vi "Measurement UI.vi"() -> ()   [LabVIEW 2021]
uses:
  bhava/source/shared/controls/PCM Interface Type_Copy.ctl
  bhava/source/shared/controls/Audio ADC Controls.lvlib
  <vilib>/PDM Acquisition Toolkit/shared/controls/Digital Edge.ctl
  <vilib>/PDM Acquisition Toolkit/shared/PDM Shared.lvlib
  bhava/source/shared/Audio ADC Shared.lvlib
panel:
  in  "MeasGraphs":T1(tab)=enum."Time Domain"
  out "FreqDomainGraph":cluster{"f0":dbl, "df":dbl, "Spectrum":dbl[]}[](graph) caption="AC"
  out "TimeDomainGraph":waveform(dbl)[](graph) caption="AC"
  out "Spectrum":dbl[](array[numeric])
  out "df":dbl[](array[numeric])
  out "f0":dbl[](array[numeric])
  out "Time domain":dbl[](array[numeric])
  out "dt":dbl[](array[numeric])
  out "t0":dbl[](array[numeric])
  out "SFDR":dbl[](array[numeric])
  out "Gain error":dbl[](array[numeric])
  out "Dynamic range":dbl[](array[numeric])
  out "THD":dbl[](array[numeric])
  out "THD+N":dbl[](array[numeric])
  out "SNR":dbl[](array[numeric])
  out "Calculated amplitude":dbl[](array[numeric])
  out "Calculated frequency":dbl[](array[numeric])
  out "MeasTable":string[][](table)
  in  "Configuration tab":enum32{"Protocol", "Measurement"}(tab)=enum."Measurement"
  in  "Endianness":enum32{"MSB First", "LSB First"}(ring)
  in  "Bit clock edge  sync":enum32{"Rising", "Falling"}(ring)=enum."Falling"
  in  "Frame sync edge for Channel 0":enum32{"Rising", "Falling"}(ring)=enum."Falling"
  in  "Channel count per frame":u32=2
  in  "Channel length":u32=32
  in  "Bit depth":u32=24
  in  "Channel 0 offset":u32=1
  in  "Data Justification":enum32{"Left Justified", "Right Justified"}(ring) caption="Data justification"
  in  "Frame length":u32=64
  in  "Frame sync pulse width":u32=32
  in  "I2S":bool
  in  "LJ":bool
  in  "RJ":bool
  in  "TDM":bool
  in  "Band stop":dbl=20000.0 format="%#.6pHz"
  in  "Band start":dbl=20.0 format="%#.6pHz"
  in  "Right channel analog source resource name":string(combo) caption="Right channel resource name"
  in  "Protocol capture resource name":string(combo) caption="Resource name"
  in  "Measurement Duration":dbl=0.1 caption="Measurement duration" format="%#_6ps"
  in  "Left channel analog source resource name":string(combo) caption="Left channel resource name"
  in  "Channel name":string
  in  "Full scale range":dbl=2.825 caption="FULL SCALE RANGE" format="%.3pV"
  in  "Weighting Filter":string(combo)="Linear" caption="Weighting filter"
  in  "Data line":u32
  in  "Sample rate":dbl=44100.0 format="%#.6pHz"
  in  "Measurement settings":string="Measurement Settings"
  in  "Amplitude":dbl=-1.0 format="%#_6pdB"
  in  "Frequency":dbl=1000.0 format="%#_6pHz"
  in  "Right acquisition channel":u32=1
  in  "Left acquisition channel":u32
  in  "Analog source":string="Analog source"
  in  "Digital capture":string="Digital capture"
  # "Protocols"
  # "PCM data configuration"
  # "Frame sync clock control"
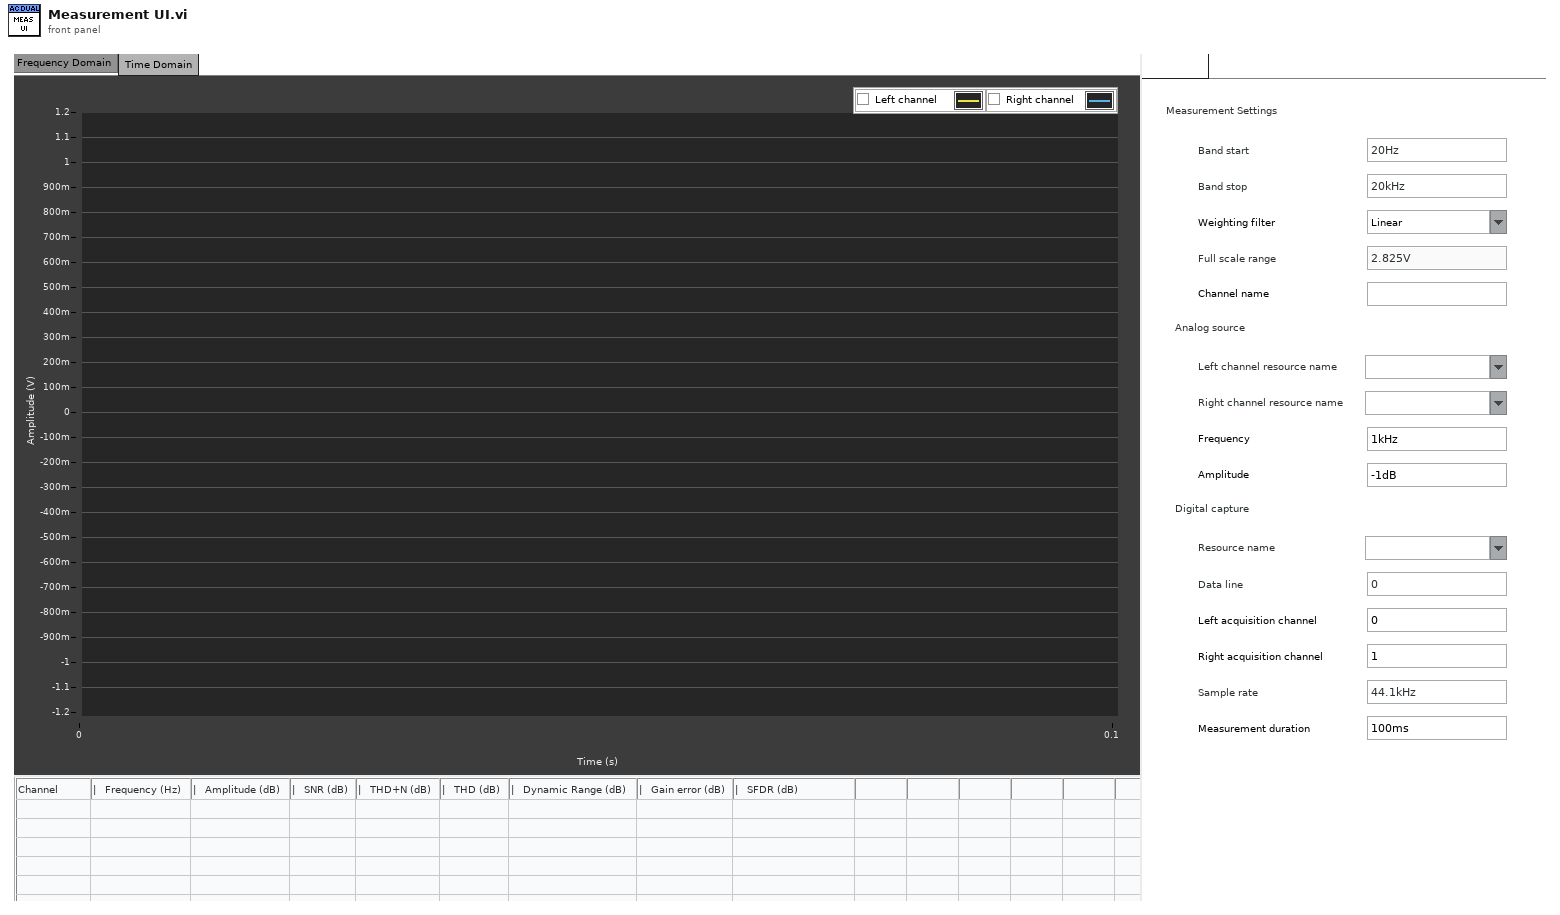
[diagram p1: front panel]
types:
  T1 = enum32{"Frequency Domain", "Time Domain", "Hidden Controls"}
  T2 = typedef "PDM Shared.lvlib/Digital Edge.ctl" = enum8{"Rising", "Falling"}
  T3 = typedef "Audio ADC Controls.lvlib/PCM Interface Type_Copy.ctl" = enum16{"I2S", "Left Justified", "Right Justified", "TDM 4 Channel", "TDM 6 Channel", "TDM 8 Channel", "DSP mode", "DSP mode with 1 bit delay", "PCM Short Frame", "PCM Long Frame"}
  T4 = typedef "PDM Shared.lvlib/PCM Frame Sync Control.ctl" = cluster{"Frame Length":u16, "Frame Sync Pulse Width":u16, "Bit Clock Edge  Sync":T2}
  T5 = typedef "PDM Shared.lvlib/PCM Data Format Configuration.ctl" = cluster{"Frame Sync Edge for Channel 0":T2, "Channel Count Per Frame":u8, "Channel Length":u16, "Bit Depth":u8, "Channel 0 Offset":u16, "Endianness":T6, "Data Justification":T7}
  T6 = typedef "PDM Shared.lvlib/PCM Bit Endianness.ctl" = enum16{"MSB First", "LSB First"}
  T7 = typedef "PDM Shared.lvlib/PCM Data Justification.ctl" = enum16{"Left Justified", "Right Justified"}
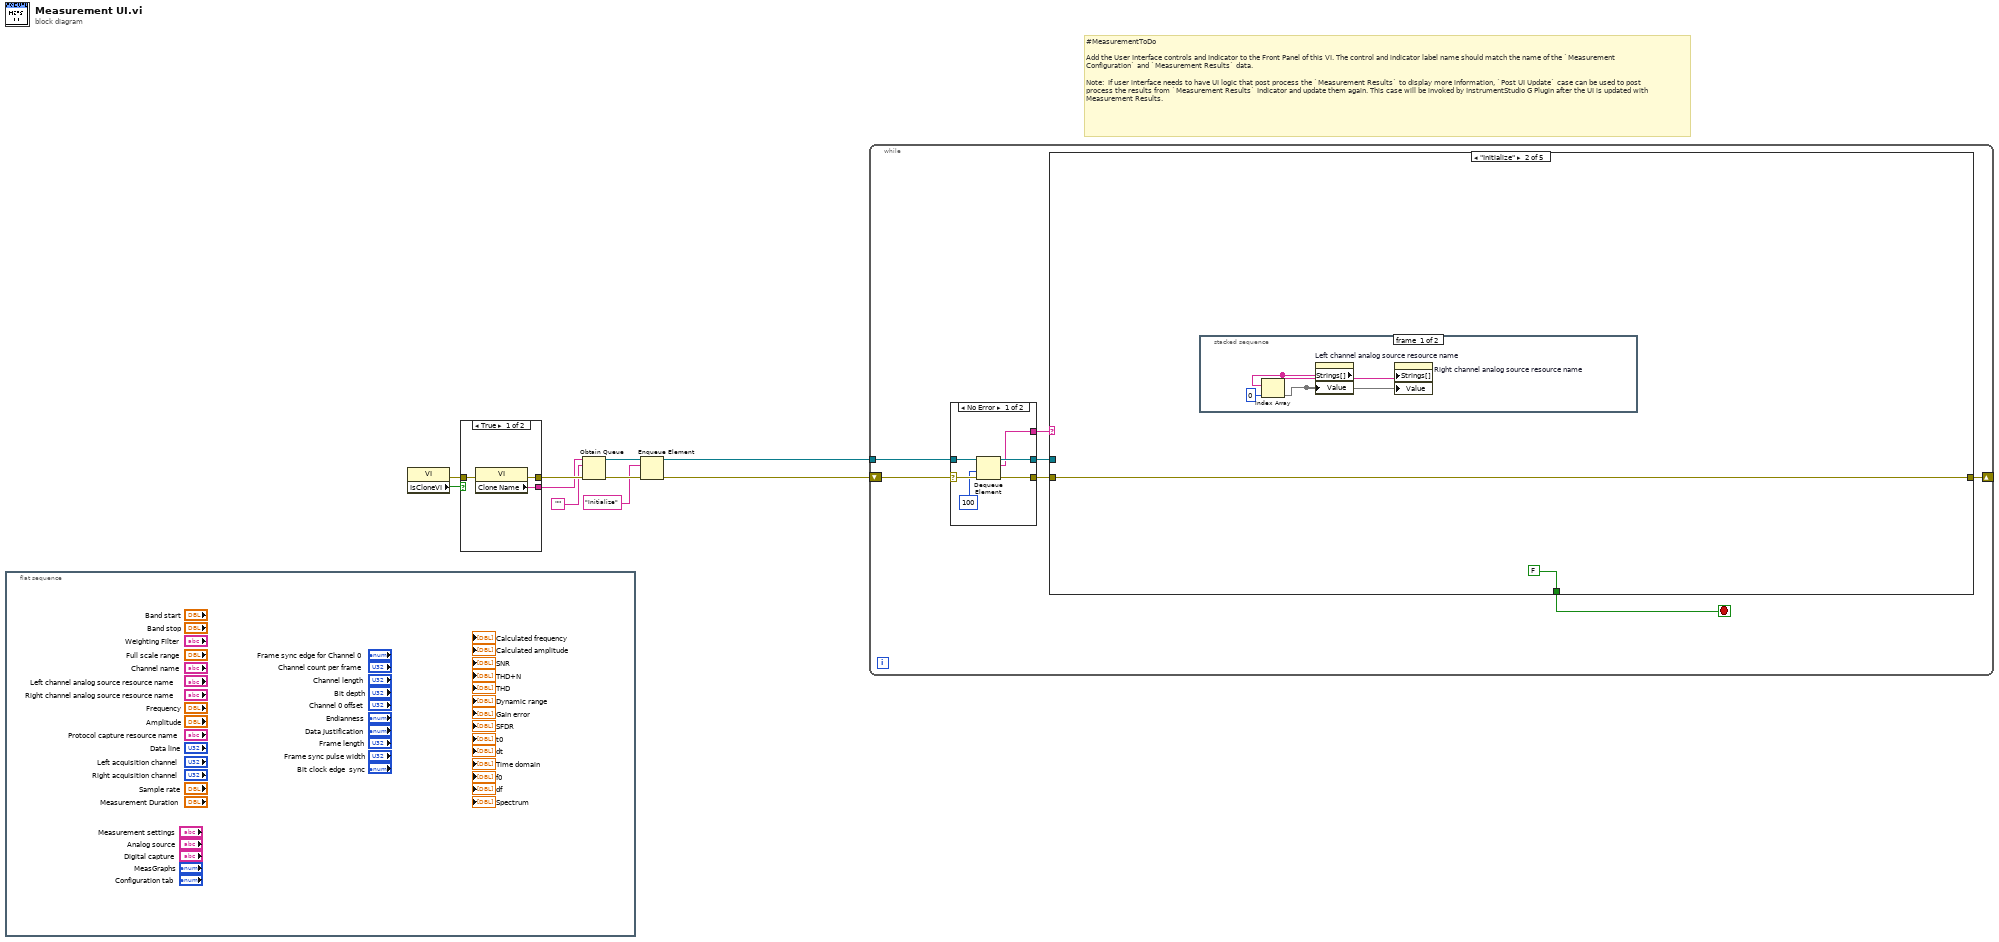
[diagram p0: block diagram]
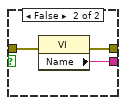
[diagram p2: hidden frame]
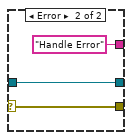
[diagram p3: hidden frame]
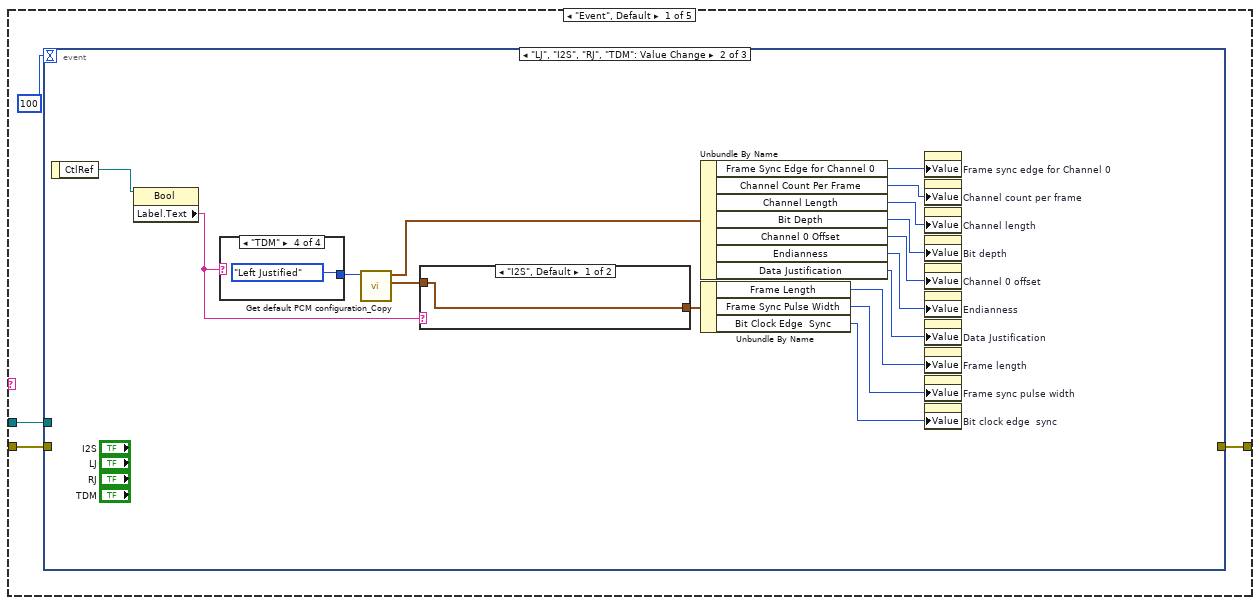
[diagram p4: hidden frame]
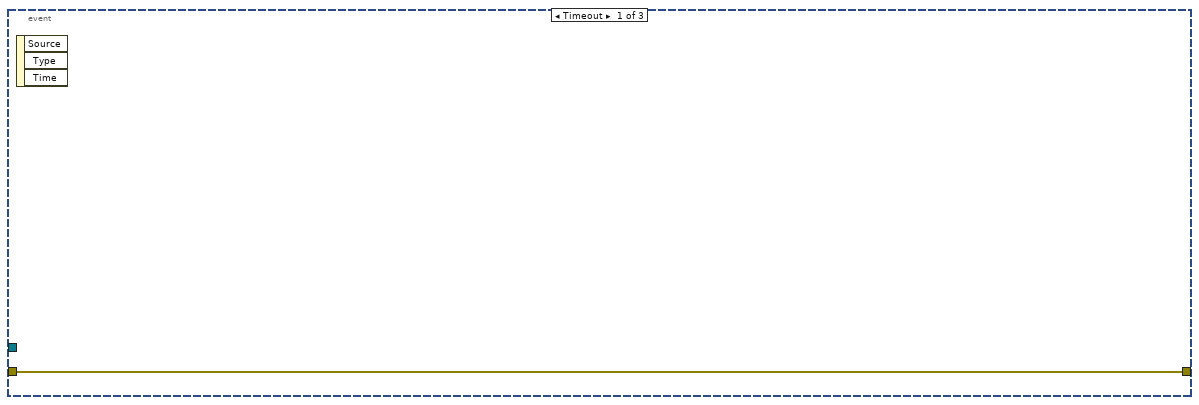
[diagram p5: hidden frame]
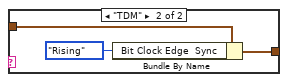
[diagram p6: hidden frame]
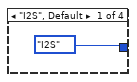
[diagram p7: hidden frame]
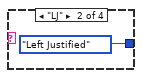
[diagram p8: hidden frame]
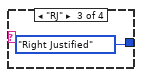
[diagram p9: hidden frame]
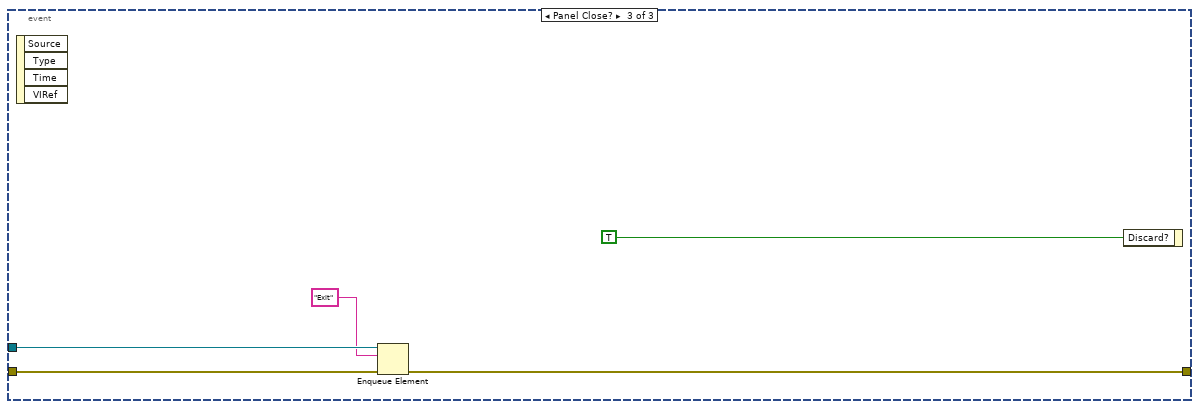
[diagram p10: hidden frame]
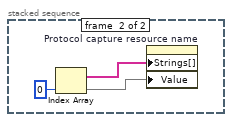
[diagram p11: hidden frame]
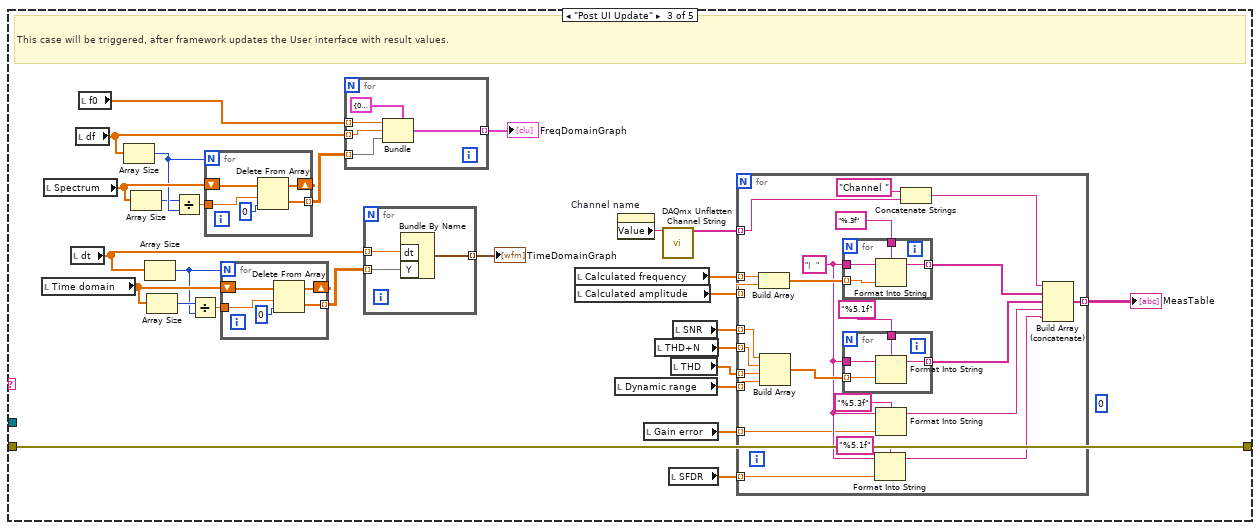
[diagram p12: hidden frame]
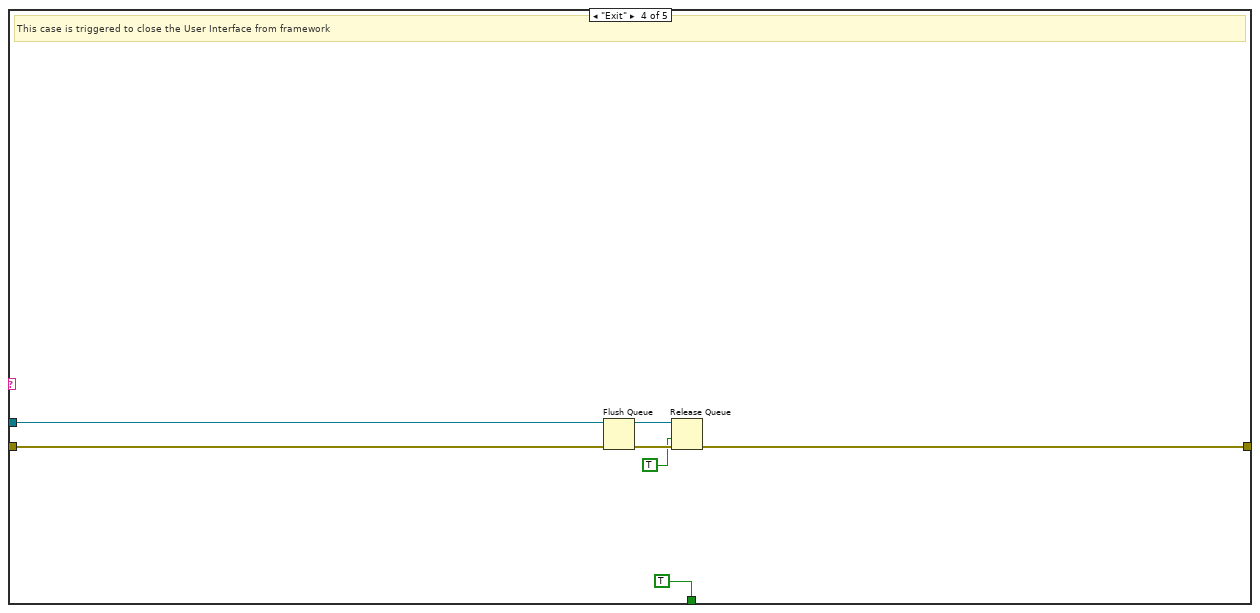
[diagram p13: hidden frame]
diagram:
  # "#MeasurementToDo  \n\nAdd the User Interface controls and Indicator to the Front Panel of this VI. The control and indicator label name should match the name of the `Measurement Configuration` and `Measurement Results` data.\n\nNote:  If user interface needs to have UI logic that post process the `Measurement Results` to display more information, `Post UI Update` case can be used to post process the results from `Measurement Results` Indicator and update them again. This case will be invoked by InstrumentStudio G Plugin after the UI is updated with Measurement Results."
  n1 = flat-sequence {
    frame #0 {
    }
  }
  n2 = property class="VI"() -> (error out=w1:errorcluster, "IsCloneVI"=w2:bool)  [unwired: 2 in, 1 out]
  n3 = case shown="True" w2 {
    tunnel: [w13 w16] -> w10
    tunnel: [w12 w15] -> w9
    tunnel: w1 -> [w11 w14]
    frame True {
      n4 = property class="VI"(error in=w11) -> (error out=w13:errorcluster, "Clone Name"=w12:string)  [unwired: 1 in, 1 out]
    }
    frame False {
      n5 = property class="VI"(error in=w14) -> (error out=w16:errorcluster, "Name"=w15:string)  [unwired: 1 in, 1 out]
    }
  }
  n6 = Obtain Queue(name (unnamed)=w9, element data type="", error in (no error)=w10) -> (queue out=w6:refnum<queue>, error out=w8:errorcluster)  [unwired: 2 in, 1 out]
  n7 = Enqueue Element(queue=w6, element="Initialize", error in (no error)=w8) -> (queue out=w5:refnum<queue>, error out=w7:errorcluster)  [unwired: 1 in, 1 out]
  n8 = while {
    shift-right: [w18] -> _
    shift-left: w7 -> [w23]
    tunnel: w5 -> [w21]
    stop <- w17 stop-if-true
    n9 = case shown="No Error" w23 {
      selector: w23 -> [w29 w32]
      tunnel: [w28 w32] -> w22
      tunnel: w21 -> [w27 w31]
      tunnel: [w26 w31] -> w20
      tunnel: [w25 "Handle Error"] -> w19
      frame No Error {
        n10 = Dequeue Element(queue=w27, timeout in ms (-1)=100, error in (no error)=w29) -> (queue out=w26:refnum<queue>, element=w25:string, error out=w28:errorcluster)  [unwired: 1 out]
      }
      frame Error {
      }
    }
    n11 = case shown="\"Initialize\"" w19 {
      tunnel: w22 -> [w35 w68 w101 w157 w158]
      tunnel: w20 -> [w33 _ _ w155 _]
      tunnel: [w36 w68 w101 w152 w158] -> w18
      tunnel: [_ FALSE _ TRUE _] -> w17
      frame "Event", Default {
        n12 = event shown="[1] \"LJ\", \"I2S\", \"RJ\", \"TDM\": Value Change" {
          selector: _ -> [_ _ _]
          dyn-events: _ -> [_ _ _]
          timeout: 100 -> [_ _ _]
          tunnel: [w37 _ w64] -> w36
          tunnel: w35 -> [w37 _ w65]
          tunnel: w33 -> [_ _ w63]
          event Timeout {
            n13 = event-data() -> ()  [unwired: 1 in, 3 out]
          }
          event "LJ", "I2S", "RJ", "TDM": Value Change {
            n14 = event-data() -> ("CtlRef"=w38:refnum<vi>)  [unwired: 1 in]
            n15 = property class="Bool"(reference=w38) -> ("Label.Text"=w53:string)  [unwired: 1 in, 2 out]
            n16 = case shown="\"TDM\"" w53 {
              tunnel: [PCM_Interface_Type_Copy."I2S" ("PCM Interfaces") PCM_Interface_Type_Copy."Left Justified" ("PCM Interfaces") PCM_Interface_Type_Copy."Right Justified" ("PCM Interfaces") PCM_Interface_Type_Copy."Left Justified" ("PCM Interfaces")] -> w43
              frame "I2S", Default {
              }
              frame "LJ" {
              }
              frame "RJ" {
              }
              frame "TDM" {
              }
            }
            n17 = call "Get default PCM configuration_Copy.vi"("PCM Interfaces"=w43) -> ("Frame Sync Clock Control"=w41:T4, "PCM Data Configuration"=w42:T5)  [unwired: 9 in]
            n18 = case shown="\"I2S\", Default" w53 {
              tunnel: [w54 w56] -> w52
              tunnel: w41 -> [w54 w55]
              frame "I2S", Default {
              }
              frame "TDM" {
                n19 = Bundle By Name(cluster=w55, "Bit Clock Edge  Sync"=Digital_Edge."Rising") -> (w56:T4)
              }
            }
            n20 = Unbundle By Name(w42) -> ("Frame Sync Edge for Channel 0"=w51:T2, "Channel Count Per Frame"=w50:u8, "Channel Length"=w49:u16, "Bit Depth"=w48:u8, "Channel 0 Offset"=w47:u16, "Endianness"=w39:T6, "Data Justification"=w44:T7)
            n21 = Unbundle By Name(w52) -> ("Frame Length"=w46:u16, "Frame Sync Pulse Width"=w45:u16, "Bit Clock Edge  Sync"=w40:T2)
            n22 = property on="Frame sync edge for Channel 0" class="Enum (strict)"("Value"=w51) -> ()  [unwired: 2 in, 2 out]
            n23 = property on="Channel count per frame" class="DigNum (strict)"("Value"=w50) -> ()  [unwired: 2 in, 2 out]
            n24 = property on="Channel length" class="DigNum (strict)"("Value"=w49) -> ()  [unwired: 2 in, 2 out]
            n25 = property on="Bit depth" class="DigNum (strict)"("Value"=w48) -> ()  [unwired: 2 in, 2 out]
            n26 = property on="Channel 0 offset" class="DigNum (strict)"("Value"=w47) -> ()  [unwired: 2 in, 2 out]
            n27 = property on="Endianness" class="Enum (strict)"("Value"=w39) -> ()  [unwired: 2 in, 2 out]
            n28 = property on="Data Justification" class="Enum (strict)"("Value"=w44) -> ()  [unwired: 2 in, 2 out]
            n29 = property on="Frame length" class="DigNum (strict)"("Value"=w46) -> ()  [unwired: 2 in, 2 out]
            n30 = property on="Frame sync pulse width" class="DigNum (strict)"("Value"=w45) -> ()  [unwired: 2 in, 2 out]
            n31 = property on="Bit clock edge  sync" class="Enum (strict)"("Value"=w40) -> ()  [unwired: 2 in, 2 out]
          }
          event Panel Close? {
            n32 = event-data() -> ()  [unwired: 1 in, 4 out]
            n33 = Enqueue Element(queue=w63, element="Exit", error in (no error)=w65) -> (error out=w64:errorcluster)  [unwired: 1 in, 2 out]
            n34 = event-data("Discard?"=TRUE) -> ()  [unwired: 1 in, 1 out]
          }
        }
      }
      frame "Initialize" {
        n35 = stacked-sequence {
          frame #0 {
            n36 = Index Array(array=w70, index=0) -> (element=w69)
            n37 = property on="Left channel analog source resource name" class="CmbBox"("Value"=w69) -> ("Strings[]"=w70:string[])  [unwired: 2 in, 2 out]
            n38 = property on="Right channel analog source resource name" class="CmbBox"("Strings[]"=w70, "Value"=w69) -> ()  [unwired: 2 in, 2 out]
          }
          frame #1 {
            n39 = Index Array(index=0) -> (array=w73:string[], element=w72)
            n40 = property on="Protocol capture resource name" class="CmbBox"("Strings[]"=w73, "Value"=w72) -> ()  [unwired: 2 in, 2 out]
          }
        }
      }
      frame "Post UI Update" {
        (unwired) 0 ("disabled index (col)")
        # "This case will be triggered, after framework updates the User interface with result values."
        n41 = local read "Time domain"() -> (w98:dbl[])
        n42 = local read "Spectrum"() -> (w93:dbl[])
        n43 = local read "dt"() -> (w99:dbl[])
        n44 = local read "df"() -> (w92:dbl[])
        n45 = local read "f0"() -> (w88:dbl[])
        n46 = Array Size(array=w92) -> (size(s)=w91:i32)
        n47 = Array Size(array=w93) -> (size(s)=w89:i32)
        n48 = Array Size(array=w99) -> (size(s)=w95:i32)
        n49 = Array Size(array=w98) -> (size(s)=w97:i32)
        n50 = Divide(x=w89, y=w91) -> (x/y=w90:dbl)
        n51 = Divide(x=w97, y=w95) -> (x/y=w96:dbl)
        n52 = for {
          N: w91 -> [_]
          tunnel: w90 -> [w142]
          tunnel: [w143] -> w94 mode=indexing
          shift-right: [w144] -> _
          shift-left: w93 -> [w145]
          n53 = Delete From Array(array=w145, length=w142, index=0) -> (deleted portion=w143:dbl[], array with subset deleted=w144:dbl[])
        }
        n54 = for {
          N: w95 -> [_]
          tunnel: w96 -> [w137]
          tunnel: [w138] -> w100 mode=indexing
          shift-right: [w139] -> _
          shift-left: w98 -> [w140]
          n55 = Delete From Array(array=w140, length=w137, index=0) -> (deleted portion=w138:dbl[], array with subset deleted=w139:dbl[])
        }
        n56 = for {
          tunnel: w94 -> [w149] mode=indexing
          tunnel: [w148] -> w86 mode=indexing
          tunnel: w88 -> [w147] mode=indexing
          tunnel: w92 -> [w146] mode=indexing
          n57 = Bundle(cluster=cluster{"x0":dbl, "dx":dbl, "magnitude":dbl[]} {"x0"=0.0, "dx"=0.0, "magnitude"=[]} ("FreqDomainGraph"), "x0"=w147, "dx"=w146, "magnitude"=w149) -> (w148:cluster{"x0":dbl, "dx":dbl, "magnitude":dbl[]})
        }
        "FreqDomainGraph" <- w86
        n58 = for {
          tunnel: w99 -> [w135] mode=indexing
          tunnel: w100 -> [w134] mode=indexing
          tunnel: [w133] -> w87 mode=indexing
          n59 = Bundle By Name("dt"=w135, "Y"=w134) -> (w133:waveform(dbl))  [unwired: 1 in]
        }
        "TimeDomainGraph" <- w87
        n60 = local read "Calculated frequency"() -> (w82:dbl[])
        n61 = local read "Calculated amplitude"() -> (w81:dbl[])
        n62 = local read "Dynamic range"() -> (w83:dbl[])
        n63 = property on="Channel name" class="Str"() -> ("Value"=w77:string)  [unwired: 2 in, 2 out]
        n64 = local read "Gain error"() -> (w79:dbl[])
        n65 = local read "THD+N"() -> (w84:dbl[])
        n66 = call <vilib>:"DAQmx Unflatten Channel String.vi"("names in"=w77) -> ("names out"=w76:string[])  [unwired: 13 in, 1 out]
        n67 = local read "SFDR"() -> (w78:dbl[])
        n68 = local read "THD"() -> (w85:dbl[])
        n69 = local read "SNR"() -> (w80:dbl[])
        n70 = for {
          tunnel: w85 -> [w124] mode=indexing
          tunnel: w84 -> [w123] mode=indexing
          tunnel: w83 -> [w122] mode=indexing
          tunnel: [w115] -> w75 mode=indexing
          tunnel: w82 -> [w114] mode=indexing
          tunnel: w81 -> [w113] mode=indexing
          tunnel: w80 -> [w112] mode=indexing
          tunnel: w79 -> [w110] mode=indexing
          tunnel: w78 -> [w109] mode=indexing
          tunnel: w76 -> [w104] mode=indexing
          w111 = "|   " ("initial string")
          n71 = Build Array(w114, w113) -> (w119:dbl[])
          n72 = Build Array(w112, w123, w124, w122) -> (w118:dbl[])
          n73 = for {
            tunnel: w119 -> [w129] mode=indexing
            tunnel: w111 -> [w130]
            tunnel: "%.3f" ("initial string") -> [w131]
            tunnel: [w132] -> w117 mode=indexing
            n74 = Format Into String(format string=w131, initial string=w130, w129) -> (resulting string=w132:string)  [unwired: 1 in, 1 out]
          }
          n75 = for {
            tunnel: w118 -> [w125] mode=indexing
            tunnel: w111 -> [w126]
            tunnel: "%5.1f" ("initial string") -> [w127]
            tunnel: [w128] -> w116 mode=indexing
            n76 = Format Into String(format string=w127, initial string=w126, w125) -> (resulting string=w128:string)  [unwired: 1 in, 1 out]
          }
          n77 = Format Into String(format string="%5.1f" ("initial string"), initial string=w111, w109) -> (resulting string=w107:string)  [unwired: 1 in, 1 out]
          n78 = Format Into String(format string="%5.3f" ("initial string"), initial string=w111, w110) -> (resulting string=w108:string)  [unwired: 1 in, 1 out]
          n79 = Concatenate Strings("Channel " ("string"), w104) -> (w103:string)
          n80 = Build Array (concatenate)(w103, w117, w116, w108, w107) -> (w115:string[])
        }
        "MeasTable" <- w75
      }
      frame "Exit" {
        # "This case is triggered to close the User Interface from framework"
        n81 = Flush Queue(queue=w155, error in (no error)=w157) -> (queue out=w154:refnum<queue>, error out=w153:errorcluster)  [unwired: 1 out]
        n82 = Release Queue(queue=w154, force destroy? (F)=TRUE, error in (no error)=w153) -> (error out=w152:errorcluster)  [unwired: 2 out]
      }
      frame "Handle Error" {
      }
    }
  }
